vi "Channel_WriteLogChannel.vi"(0 "Channel in":refnum<class "Channel.lvclass">, 1 "Time":timestamp, 4 "dt per loop":dbl, 5 "error in (no error)":errorcluster, 6 "Group Name":string, 7 "Loop Counter":i32, 8 "tdms file":refnum<k34>) -> (14 "Channel out":refnum<class "Channel.lvclass">, 15 "tdms file out":refnum<k34>, 19 "error out":errorcluster)   [LabVIEW 2023, in "Channel.lvclass"]
doc: "Write the channel to file if the current decimation set and loop iteration are divisible with one another."
uses:
  Channel.lvclass
  Channel.lvclass/Channel.ctl
panel:
  out "output waveform":waveform(dbl)
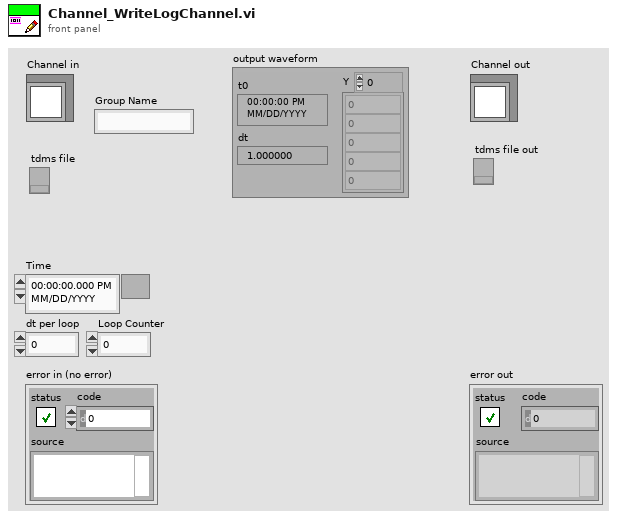
[diagram p1: front panel]
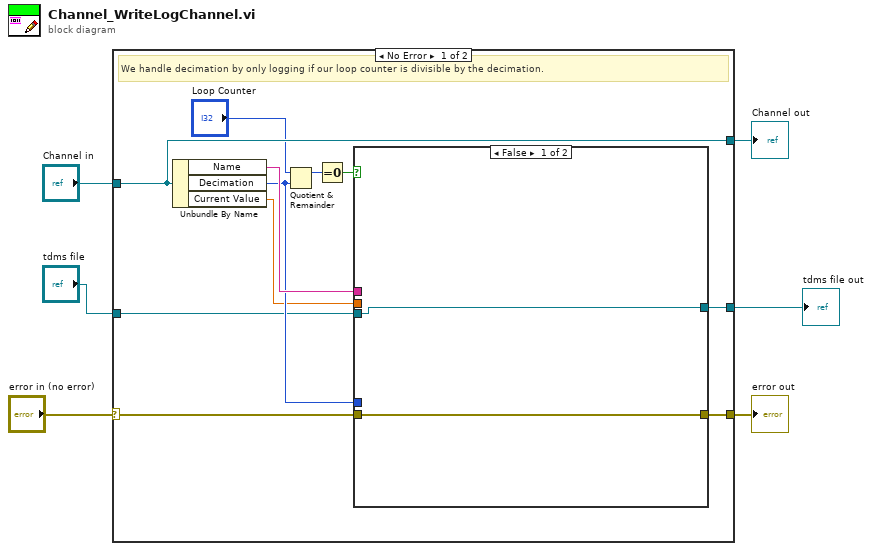
[diagram p0: block diagram]
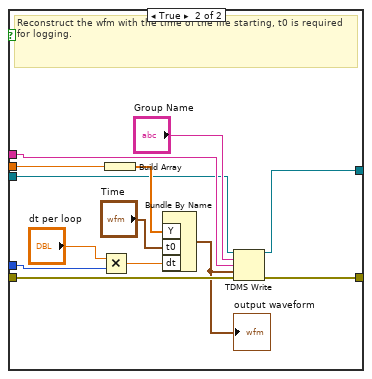
[diagram p2: hidden frame]
diagram:
  n1 = case shown="No Error" "error in (no error)" {
    selector: "error in (no error)" -> [w12 w35]
    tunnel: [w13 w35] -> w5
    tunnel: [w11 w34] -> w3
    tunnel: "Channel in" -> [w11 w34]
    tunnel: "tdms file" -> [w8 w33]
    tunnel: [w7 w33] -> w1
    frame No Error {
      # "We handle decimation by only logging if our loop counter is divisible by the decimation."
      n2 = Unbundle By Name(w11) -> ("Name"=w17:string, "Decimation"=w15:i32, "Current Value"=w9:dbl)
      n3 = Quotient & Remainder(x="Loop Counter", y=w15) -> (x-y*floor(x/y)=w16:i32)  [unwired: 1 out]
      n4 = Equal To 0?(x=w16) -> (x = 0?=w14:bool)
      n5 = case shown="False" w14 {
        tunnel: w17 -> [_ w31]
        tunnel: w15 -> [_ w25]
        tunnel: w12 -> [w19 w30]
        tunnel: [w19 w29] -> w13
        tunnel: w9 -> [_ w22]
        tunnel: w8 -> [w18 w21]
        tunnel: [w18 w20] -> w7
        frame False {
        }
        frame True {
          # "Reconstruct the wfm with the time of the file starting, t0 is required for logging."
          n6 = Multiply(x="dt per loop", y=w25) -> (x*y=w26:dbl)
          n7 = Build Array(w22) -> (w28:dbl[])
          n8 = Bundle By Name("Y"=w28, "t0"="Time", "dt"=w26) -> (w27:waveform(dbl))  [unwired: 1 in]
          "output waveform" <- w27
          n9 = TDMS Write(0:w21, 5:"Group Name", 7:w31, 9:w27, 11:w30) -> (4:w20:refnum<k34>, 15:w29:errorcluster)  [unwired: 1 in, 2 out]
        }
      }
    }
    frame Error {
    }
  }
  "error out" <- w5
  "Channel out" <- w3
  "tdms file out" <- w1
